vi "cal scope.vi"(9 "Channel Name":string="0,1,2,3", 10 "scope cal data":T2(array[cluster]), 11 "measured data":T1(array[cluster])) -> (3 "measured and cal data":T1(array[cluster]))   [LabVIEW 2021]
uses:
  <vilib>/Analysis/1siggen.llb/Ramp Pattern by Delta.vi
  <vilib>/Analysis/NI_AALBase.lvlib
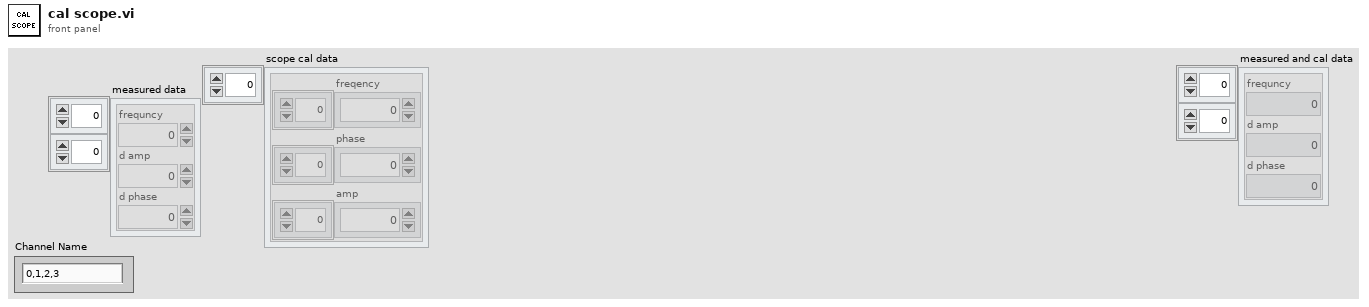
[diagram p1: front panel]
types:
  T1 = cluster{"frequncy":dbl, "d amp":dbl, "d phase":dbl}[][]
  T2 = cluster{"freqency":dbl[], "phase":dbl[], "amp":dbl[]}[]
  T3 = cluster{"freqency":dbl[], "phase":dbl[], "amp":dbl[]}
  T4 = cluster{"frequncy":dbl, "d amp":dbl, "d phase":dbl}
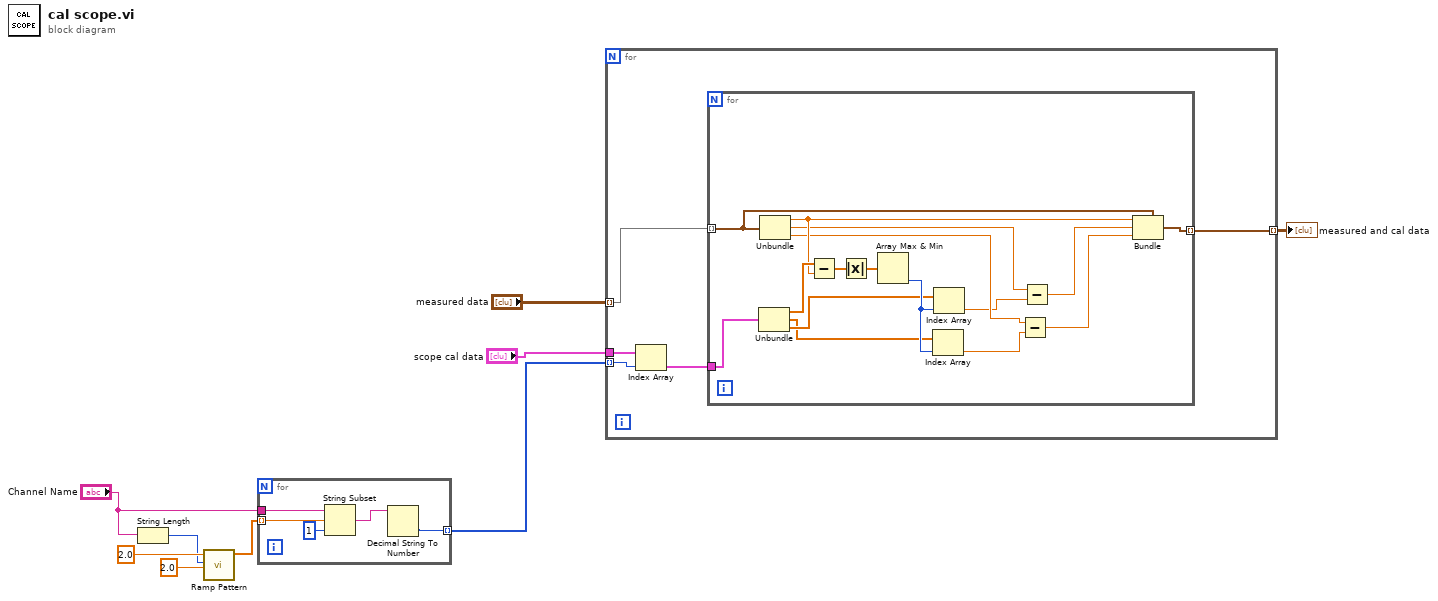
[diagram p0: block diagram]
diagram:
  n1 = String Length(string="Channel Name") -> (length=w8:i32)
  n2 = call-poly <vilib>:"Ramp Pattern.vi"("start"=2.0, "end"=w8, "delta"=2.0) -> ("Ramp Pattern"=w6:dbl[])  [unwired: 6 in, 2 out]
  n3 = for {
    tunnel: w6 -> [w14] mode=indexing
    tunnel: "Channel Name" -> [w12]
    tunnel: [w10] -> w2 mode=indexing
    n4 = String Subset(string=w12, offset (0)=w14, length (rest)=1 ("length (rest)")) -> (substring=w11:string)
    n5 = Decimal String To Number(string=w11) -> (number=w10:i32)  [unwired: 2 in, 1 out]
  }
  n6 = for {
    tunnel: "measured data" -> [w17] mode=indexing
    tunnel: "scope cal data" -> [w19]
    tunnel: w2 -> [w18] mode=indexing
    tunnel: [w15] -> w1 mode=indexing
    n7 = Index Array(array=w19, index=w18) -> (element=w16:T3)
    n8 = for {
      tunnel: w17 -> [w31] mode=indexing
      tunnel: w16 -> [w35]
      tunnel: [w22] -> w15 mode=indexing
      n9 = Unbundle(w35) -> ("freqency"=w34:dbl[], "phase"=w20:dbl[], "amp"=w21:dbl[])
      n10 = Unbundle(w31) -> ("frequncy"=w30:dbl, "d amp"=w28:dbl, "d phase"=w27:dbl)
      n11 = Subtract(x=w34, y=w30) -> (x-y=w33:dbl[])
      n12 = Absolute Value(x=w33) -> (abs(x)=w32:dbl[])
      n13 = Array Max & Min(array=w32) -> (min index (indices)=w29:i32)  [unwired: 3 out]
      n14 = Index Array(array=w20, index=w29) -> (element=w25:dbl)
      n15 = Index Array(array=w21, index=w29) -> (element=w26:dbl)
      n16 = Subtract(x=w27, y=w25) -> (x-y=w23:dbl)
      n17 = Subtract(x=w28, y=w26) -> (x-y=w24:dbl)
      n18 = Bundle(cluster=w31, "frequncy"=w30, "d amp"=w24, "d phase"=w23) -> (w22:T4)
    }
  }
  "measured and cal data" <- w1
